vi "Sub_SetStrobeProfile.vi"(0 "Step":u32, 1 "Device Handle":u32, 2 "Channel":i32, 3 "Tset":u32, 4 "Iset":u32) -> ()   [LabVIEW 2013]
uses:
  documentation/SDK/x64_lib/Mightex_LEDDriver_SDK.dll
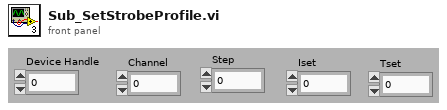
[diagram p1: front panel]
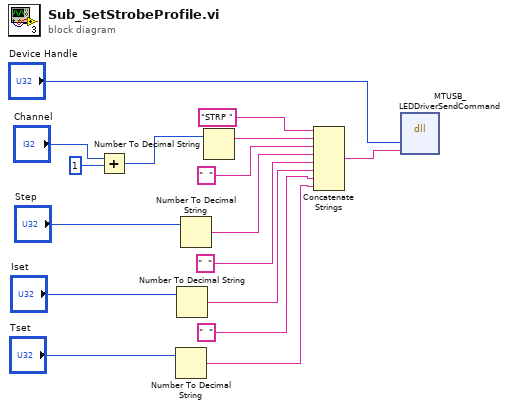
[diagram p0: block diagram]
diagram:
  n1 = Add(x="Channel", y=1) -> (x+y=w1:i32)
  n2 = Number To Decimal String(number="Tset") -> (decimal integer string=w4:string)  [unwired: 1 in]
  n3 = Number To Decimal String(number="Iset") -> (decimal integer string=w12:string)  [unwired: 1 in]
  n4 = Number To Decimal String(number="Step") -> (decimal integer string=w14:string)  [unwired: 1 in]
  n5 = Number To Decimal String(number=w1) -> (decimal integer string=w8:string)  [unwired: 1 in]
  n6 = Concatenate Strings("STRP ", w8, "  ", w14, "  ", w12, "  ", w4) -> (w15:string)
  n7 = dll-call lib="C:/Users/ignacio/Desktop/Patrick's File Reader Function/led_control/documentation/SDK/x64_lib/Mightex_LEDDriver_SDK.dll" fn="MTUSB_LEDDriverSendCommand"("arg1"="Device Handle", "arg2"=w15) -> ()  [unwired: 6 in, 2 out]
